vi "AirmarFlashingCode.vi"() -> ()   [LabVIEW 2013]
doc: "Set which data to transmit at what rates for the airmar. It is saved in the EEPROM, so this is only necessary for new airmars or if one gets wiped accidentally."
panel:
  in  "VISA Refnum in":refnum<visa-resource-name>
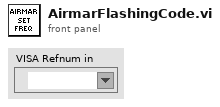
[diagram p1: front panel]
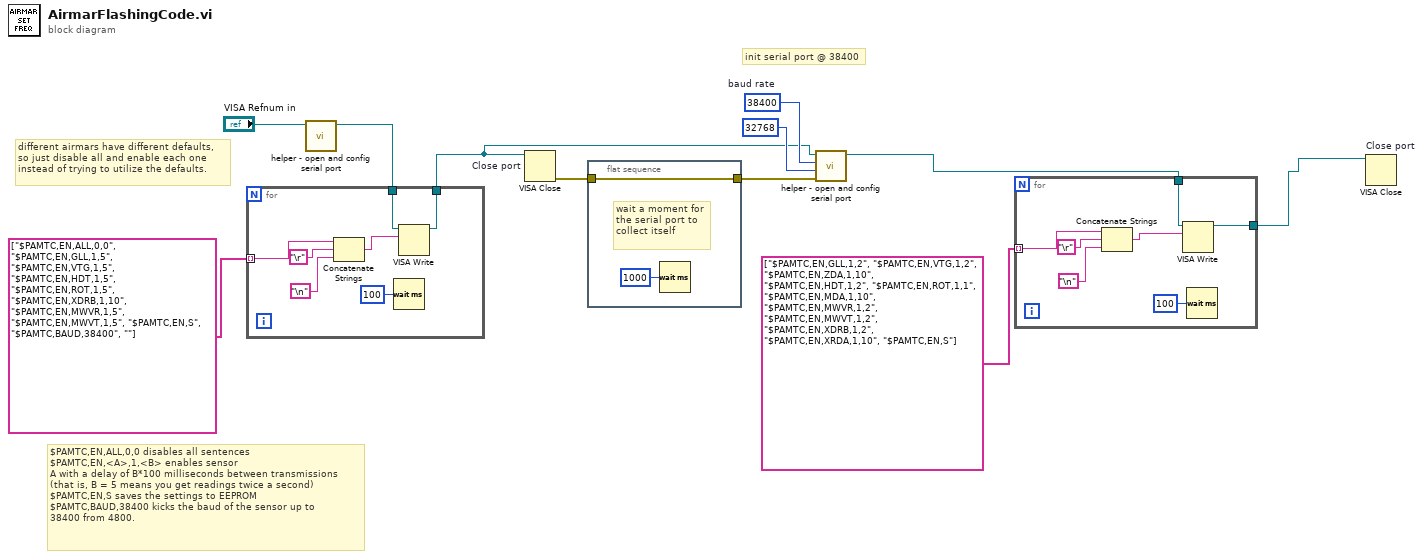
[diagram p0: block diagram]
diagram:
  w9 = u32 38400  # baud rate
  # "$PAMTC,EN,ALL,0,0 disables all sentences\n$PAMTC,EN,<A>,1,<B> enables sensor\nA with a delay of B*100 milliseconds between transmissions\n(that is, B = 5 means you get readings twice a second)\n$PAMTC,EN,S saves the settings to EEPROM\n$PAMTC,BAUD,38400 kicks the baud of the sensor up to\n38400 from 4800."
  # "different airmars have different defaults,\nso just disable all and enable each one\ninstead of trying to utilize the defaults."
  # "init serial port @ 38400"
  n1 = call "helper - open and config serial port.vi"("VISA Refnum in"="VISA Refnum in") -> ("VISA Refnum out"=w4:refnum<visa-resource-name>)  [unwired: 9 in, 1 out]
  n2 = for {
    tunnel: string[] ["$PAMTC,EN,ALL,0,0", "$PAMTC,EN,GLL,1,5", "$PAMTC,EN,VTG,1,5", "$PAMTC,EN,HDT,1,5", "$PAMTC,EN,ROT,1,5", "$PAMTC,EN,XDRB,1,10", "$PAMTC,EN,MWVR,1,5", "$PAMTC,EN,MWVT,1,5", "$PAMTC,EN,S", "$PAMTC,BAUD,38400", ""] ("4800 Baud Commands") -> [w16] mode=indexing
    tunnel: w4 -> [w14]
    tunnel: [w12] -> w3
    n3 = Concatenate Strings(w16, "\r", "\n") -> (w15:string)
    n4 = Wait (ms)(milliseconds to wait=u32 100) -> ()  [unwired: 1 out]
    n5 = VISA Write(VISA resource name=w14, write buffer=w15) -> (VISA resource name out=w12:refnum<visa-resource-name>)  [unwired: 1 in, 2 out]
  }
  n6 = VISA Close "Close port"(VISA resource name=w3) -> (error out=w7:errorcluster)  [unwired: 1 in]
  n7 = flat-sequence {
    tunnel: w7 -> [w19]
    tunnel: [w19] -> w6
    frame #0 {
      # "wait a moment for the serial port to collect itself"
      n8 = Wait (ms)(milliseconds to wait=u32 1000) -> ()  [unwired: 1 out]
    }
  }
  n9 = call "helper - open and config serial port.vi"("error in (no error)"=w6, "Input\nbuffer size"=u32 32768 ("Input\nbuffer size"), "baud rate"=w9, "VISA Refnum in"=w3) -> ("VISA Refnum out"=w2:refnum<visa-resource-name>)  [unwired: 6 in, 1 out]
  n10 = for {
    tunnel: string[] ["$PAMTC,EN,GLL,1,2", "$PAMTC,EN,VTG,1,2", "$PAMTC,EN,ZDA,1,10", "$PAMTC,EN,HDT,1,2", "$PAMTC,EN,ROT,1,1", "$PAMTC,EN,MDA,1,10", "$PAMTC,EN,MWVR,1,2", "$PAMTC,EN,MWVT,1,2", "$PAMTC,EN,XDRB,1,2", "$PAMTC,EN,XRDA,1,10", "$PAMTC,EN,S"] ("38400 Baud Commands") -> [w25] mode=indexing
    tunnel: w2 -> [w24]
    tunnel: [w23] -> w1
    n11 = Concatenate Strings(w25, "\r", "\n") -> (w22:string)
    n12 = VISA Write(VISA resource name=w24, write buffer=w22) -> (VISA resource name out=w23:refnum<visa-resource-name>)  [unwired: 1 in, 2 out]
    n13 = Wait (ms)(milliseconds to wait=u32 100) -> ()  [unwired: 1 out]
  }
  n14 = VISA Close "Close port"(VISA resource name=w1) -> ()  [unwired: 1 in, 1 out]
